vi "DSF.Shared.Configuration.Transfer Group.Channel Count.vi"(8 "error in (no error)":errorcluster, 11 "Transfer Group Configuration in":refnum<class "DSF.Shared.Configuration.Transfer Group.lvclass">) -> (0 "error out":errorcluster, 2 "total channel count":u64, 3 "Transfer Group Configuration out":refnum<class "DSF.Shared.Configuration.Transfer Group.lvclass">)   [LabVIEW 2017, in "DSF.Engine.lvlib" / "DSF.Shared.Configuration.Transfer Group.lvclass"]
uses:
  DSF.Shared.Configuration.Transfer Group.lvclass
  DSF.Shared.Configuration.Transfer Group.lvclass/DSF.Shared.Configuration.Transfer Group.ctl
  Transfer/DSF.Shared.Configuration.Transfer.lvclass
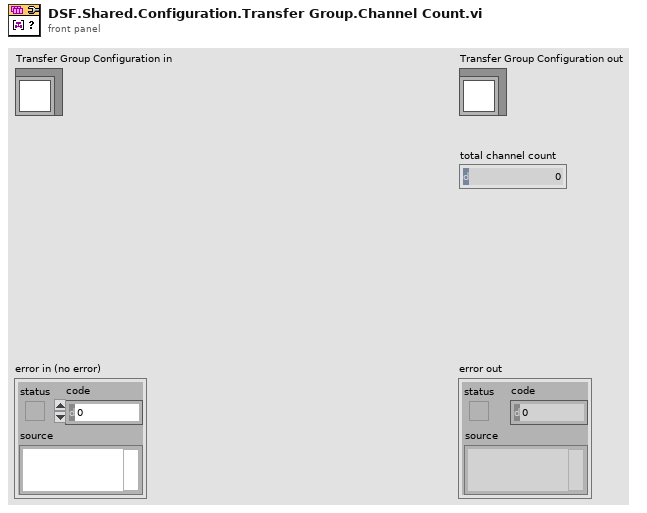
[diagram p1: front panel]
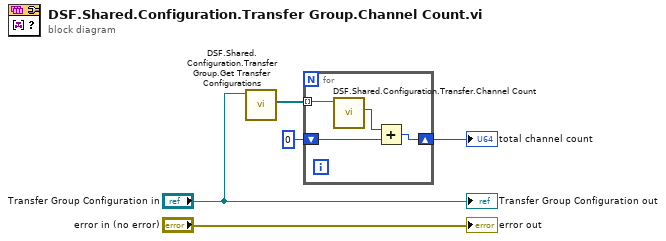
[diagram p0: block diagram]
diagram:
  n1 = call "DSF.Shared.Configuration.Transfer Group.Get Transfer Configurations.vi"("Transfer Group Configuration in"="Transfer Group Configuration in") -> ("Transfer Configurations"=w4:refnum<class "DSF.Shared.Configuration.Transfer.lvclass">[])  [unwired: 9 in, 1 out]
  n2 = for {
    tunnel: w4 -> [w7] mode=indexing
    shift-right: [w9] -> w1
    shift-left: u64 0 -> [w8]
    n3 = call "DSF.Shared.Configuration.Transfer.Channel Count.vi"("Transfer Configuration in"=w7) -> ("total channel count"=w6:u64)  [unwired: 8 in, 2 out]
    n4 = Add(x=w6, y=w8) -> (x+y=w9:u64)
  }
  "total channel count" <- w1
  "error out" <- "error in (no error)"
  "Transfer Group Configuration out" <- "Transfer Group Configuration in"
